vi "CreateFolders.vi"(8 "error in (no error)":errorcluster, 11 "baseClass in":refnum<class "baseClass.lvclass">) -> (0 "error out":errorcluster, 3 "baseClass out":refnum<class "baseClass.lvclass">)   [LabVIEW 2013, in "baseClass.lvclass"]
uses:
  baseClass.lvclass
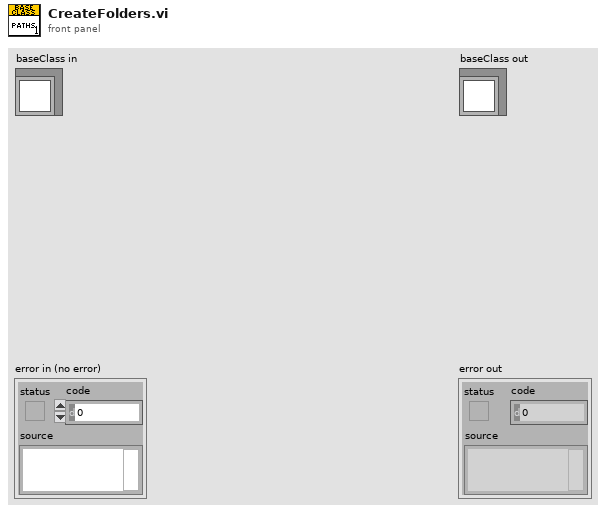
[diagram p1: front panel]
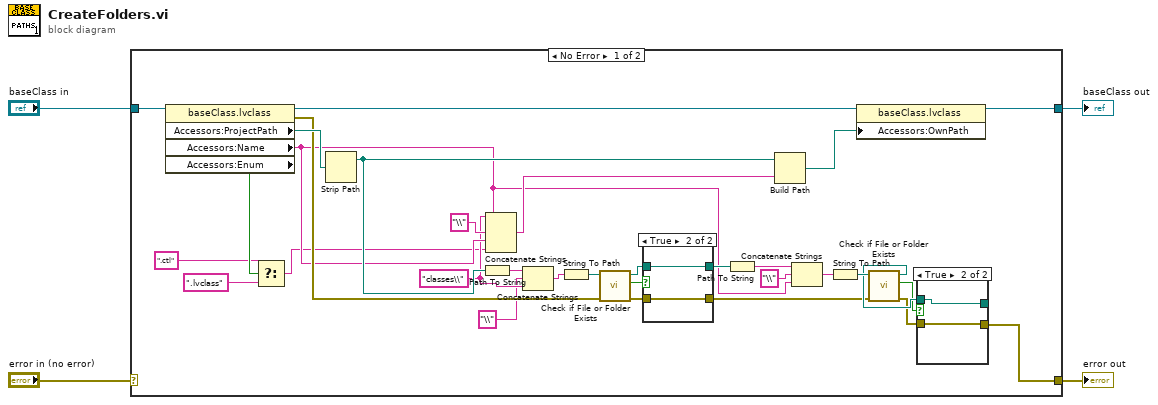
[diagram p0: block diagram]
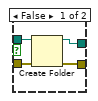
[diagram p2: hidden frame]
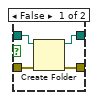
[diagram p3: hidden frame]
diagram:
  n1 = case shown="No Error" "error in (no error)" {
    selector: "error in (no error)" -> [_ w50]
    tunnel: [w19 w50] -> w3
    tunnel: [w14 w49] -> w1
    tunnel: "baseClass in" -> [w36 w49]
    frame No Error {
      w10 = "classes\\"
      n2 = property class="baseClass.lvclass"(reference=w36) -> (reference out=w35:refnum<class "baseClass.lvclass">, error out=w15:errorcluster, "Accessors:ProjectPath"=w34:path, "Accessors:Name"=w12:string, "Accessors:Enum"=w8:bool)  [unwired: 1 in]
      n3 = Select(t=".ctl", s=w8, f=".lvclass") -> (s? t:f=w6:string)
      n4 = Strip Path(path=w34) -> (stripped path=w31:path)  [unwired: 1 out]
      n5 = Path To String(path=w31) -> (string=w30:string)
      n6 = Concatenate Strings(w10, w12, "\\", w12, w6) -> (w32:string)
      n7 = Concatenate Strings(w30, "\\", w10) -> (w29:string)
      n8 = String To Path(string=w29) -> (path=w28:path)
      n9 = call <vilib>:"Check if File or Folder Exists.vi"("error in (no error)"=w15, "path"=w28) -> ("error out"=w16:errorcluster, "file or folder exists?"=w27:bool, "dup path"=w26:path)  [unwired: 7 in]
      n10 = case shown="True" w27 {
        tunnel: w26 -> [w46 w48]
        tunnel: [w45 w48] -> w25
        tunnel: [w44 w47] -> w17
        tunnel: w16 -> [w43 w47]
        frame False {
          n11 = Create Folder(path (use dialog)=w46, error in=w43) -> (created path=w45:path, error out=w44:errorcluster)  [unwired: 1 in, 1 out]
        }
        frame True {
        }
      }
      n12 = Path To String(path=w25) -> (string=w24:string)
      n13 = Build Path(base path=w31, name or relative path=w32) -> (appended path=w13:path)
      n14 = Concatenate Strings(w24, "\\", w12) -> (w23:string)
      n15 = String To Path(string=w23) -> (path=w22:path)
      n16 = property class="baseClass.lvclass"(reference=w35, "Accessors:OwnPath"=w13) -> (reference out=w14:refnum<class "baseClass.lvclass">)  [unwired: 1 in, 1 out]
      n17 = call <vilib>:"Check if File or Folder Exists.vi"("error in (no error)"=w17, "path"=w22) -> ("error out"=w18:errorcluster, "file or folder exists?"=w20:bool, "dup path"=w21:path)  [unwired: 7 in]
      n18 = case shown="True" w20 {
        tunnel: w21 -> [w40 w42]
        tunnel: [w39 w42] -> _
        tunnel: [w38 w41] -> w19
        tunnel: w18 -> [w37 w41]
        frame False {
          n19 = Create Folder(path (use dialog)=w40, error in=w37) -> (created path=w39:path, error out=w38:errorcluster)  [unwired: 1 in, 1 out]
        }
        frame True {
        }
      }
    }
    frame Error {
    }
  }
  "error out" <- w3
  "baseClass out" <- w1
